vi "WFT I2C Reset.vi"(8 "Error In":errorcluster, 11 "WaveForms Session In":T1) -> (0 "Error Out":errorcluster, 2 "ret":i32, 3 "WaveForms Session Out":T1)   [LabVIEW 2020, in "lv_waveforms_toolkit.lvlib"]
uses:
  lv_waveforms_toolkit.lvlib
  WFT Session.ctl
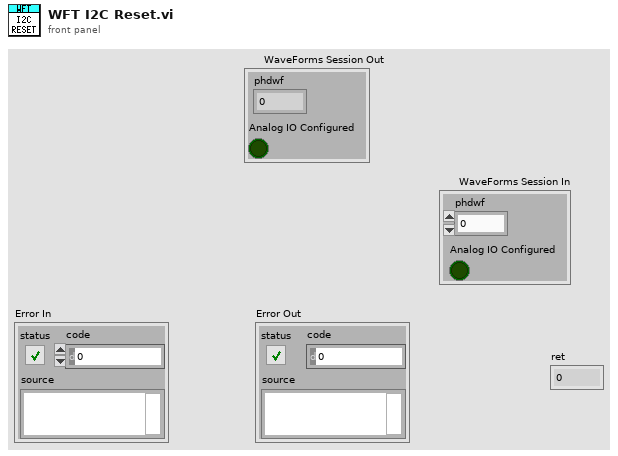
[diagram p1: front panel]
types:
  T1 = typedef "lv_waveforms_toolkit.lvlib/WFT Session.ctl" = cluster{"phdwf":i32, "Analog IO Configured":bool}
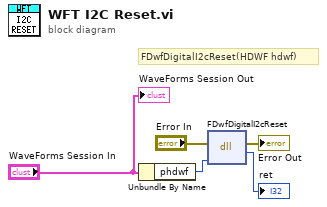
[diagram p0: block diagram]
diagram:
  # "FDwfDigitalI2cReset(HDWF hdwf)"
  n1 = Unbundle By Name("WaveForms Session In") -> ("phdwf"=w1:i32)
  n2 = dll-call lib="dwf" fn="FDwfDigitalI2cReset"(error in="Error In", "phdwf"=w1) -> (error out=→"Error Out":errorcluster, "return type"=→"ret":i32)  [unwired: 3 in, 1 out]
  "WaveForms Session Out" <- "WaveForms Session In"
